vi "interface_configure.vi"(8 "error in (no error)":errorcluster, 11 "config in":T1) -> (0 "error out":errorcluster, 3 "config out":T1)   [LabVIEW 2015, in "lv-builder-l3.lvlib"]
uses:
  lv-builder-l3.lvlib
  _controls/configuration.ctl
  <vilib>/Utility/error.llb/Error Cluster From Error Code.vi
  <vilib>/ErrorRing/Error Ring.xnode
panel:
  in  "cancel":bool
  in  "save":bool
  in  "l3_zip_file_path":path
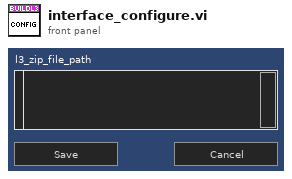
[diagram p1: front panel]
types:
  T1 = typedef "lv-builder-l3.lvlib/configuration.ctl" = cluster{"l3_archive_file_path":string}
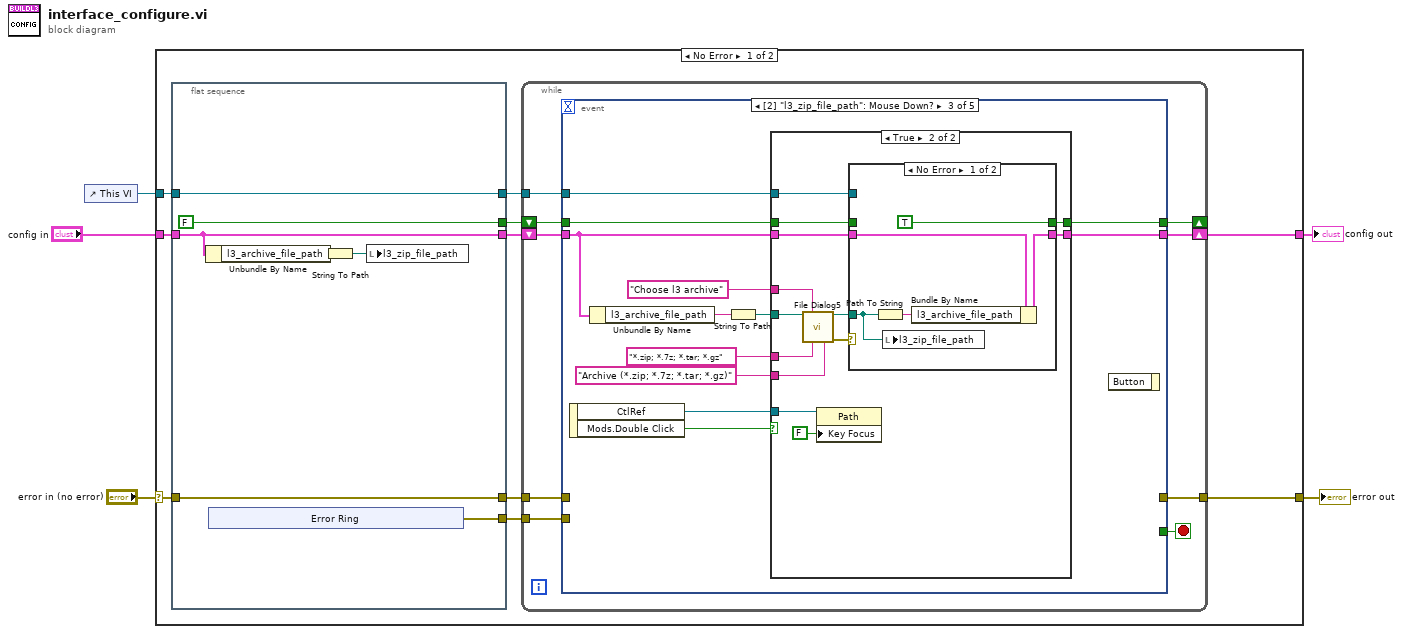
[diagram p0: block diagram]
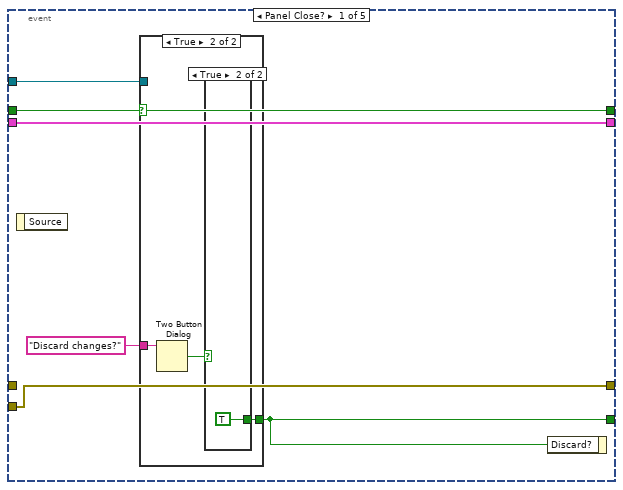
[diagram p2: hidden frame]
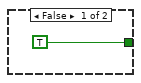
[diagram p3: hidden frame]
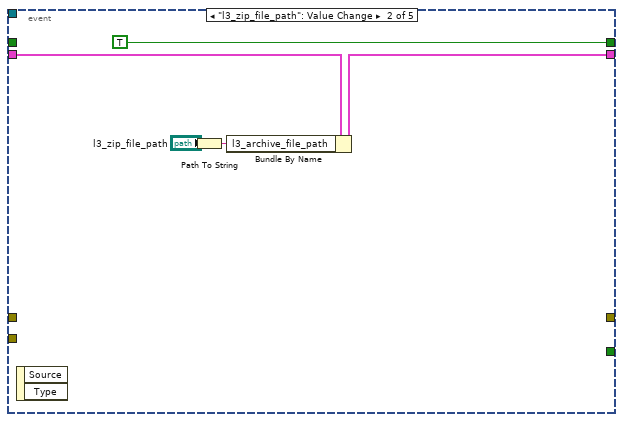
[diagram p5: hidden frame]
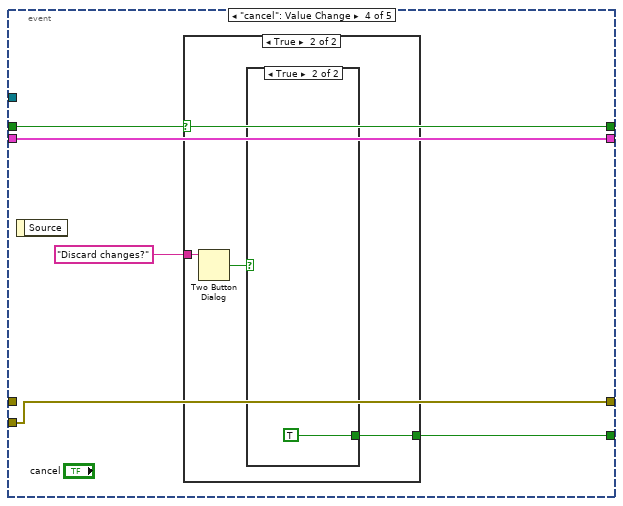
[diagram p8: hidden frame]
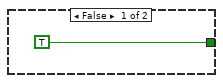
[diagram p9: hidden frame]
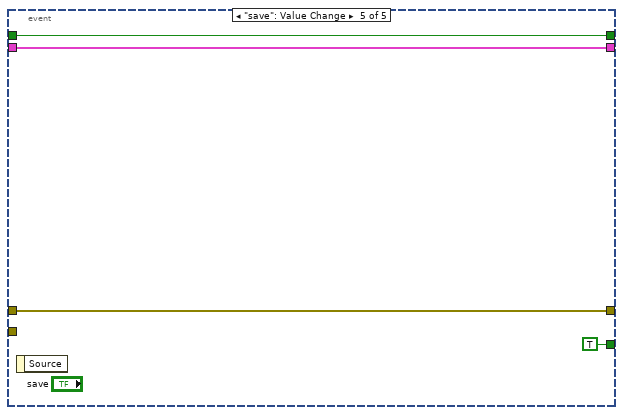
[diagram p11: hidden frame]
diagram:
  n1 = control-ref of="This VI"() -> (w3:refnum<vi>)
  n2 = case shown="No Error" "error in (no error)" {
    selector: "error in (no error)" -> [w15 w100]
    tunnel: [w9 w100] -> w4
    tunnel: w3 -> [w11 _]
    tunnel: [w8 _] -> w2
    tunnel: "config in" -> [w7 _]
    frame No Error {
      n3 = flat-sequence {
        tunnel: w15 -> [w17]
        tunnel: [w17] -> w14
        tunnel: [w18] -> w13
        tunnel: [w20] -> w12
        tunnel: w11 -> [w20]
        tunnel: [FALSE] -> w10
        tunnel: w7 -> [w18]
        tunnel: [w16] -> w6
        frame #0 {
          n4 = Unbundle By Name(w18) -> ("l3_archive_file_path"=w21:string)
          n5 = xnode "Error Ring"() -> ("error out"=w16:errorcluster)
          n6 = String To Path(string=w21) -> (path=w19:path)
          n7 = local write "l3_zip_file_path"(w19) -> ()
        }
      }
      n8 = while {
        tunnel: w14 -> [w28]
        shift-right: [w33] -> w8
        shift-left: w13 -> [w34]
        tunnel: w12 -> [w30]
        shift-right: [w31] -> _
        shift-left: w10 -> [w32]
        tunnel: [w29] -> w9
        tunnel: w6 -> [w27]
        stop <- w35 stop-if-true
        n9 = event shown="[2] \"l3_zip_file_path\": Mouse Down?" {
          selector: _ -> [_ _ _ _ _]
          dyn-events: _ -> [_ _ _ _ _]
          timeout: _ -> [_ _ _ _ _]
          tunnel: [w39 _ _ w90 TRUE ("Discard?")] -> w35
          tunnel: w30 -> [w38 _ w59 _ _]
          tunnel: w34 -> [w41 w51 w58 w89 w98]
          tunnel: [w41 w49 w61 w89 w98] -> w33
          tunnel: w32 -> [w37 _ w63 w87 w99]
          tunnel: [w37 TRUE w62 w87 w99] -> w31
          tunnel: [w36 _ _ w86 w97] -> w29
          tunnel: w28 -> [_ _ _ _ w97]
          tunnel: w27 -> [w36 _ _ w86 _]
          event Panel Close? {
            n10 = event-data() -> ()  [unwired: 1 in, 1 out]
            n11 = case shown="True" w37 {
              tunnel: [TRUE ("Discard?") w45] -> w39
              tunnel: w38 -> [_ _]
              tunnel: "Discard changes?" ("dialog_text") -> [_ w44]
              frame False {
              }
              frame True {
                n12 = Two Button Dialog(message=w44) -> (T button?=w43:bool)  [unwired: 2 in]
                n13 = case shown="True" w43 {
                  tunnel: [_ TRUE ("Discard?")] -> w45
                  frame False {
                  }
                  frame True {
                  }
                }
              }
            }
            n14 = event-data("Discard?"=w39) -> ()  [unwired: 1 in, 1 out]
          }
          event "l3_zip_file_path": Value Change {
            n15 = event-data() -> ()  [unwired: 1 in, 2 out]
            n16 = Path To String(path="l3_zip_file_path") -> (string=w47:string)
            n17 = Bundle By Name(cluster=w51, "l3_archive_file_path"=w47) -> (w49:T1)
          }
          event "l3_zip_file_path": Mouse Down? {
            n18 = event-data() -> ("CtlRef"=w54:refnum<vi>, "Mods.Double Click"=w60:bool)  [unwired: 1 in]
            n19 = Unbundle By Name(w58) -> ("l3_archive_file_path"=w57:string)
            n20 = String To Path(string=w57) -> (path=w55:path)
            n21 = case shown="True" w60 {
              tunnel: w63 -> [w65 w78]
              tunnel: w58 -> [w64 w77]
              tunnel: [w65 w76] -> w62
              tunnel: [w64 w75] -> w61
              tunnel: w59 -> [_ w74]
              tunnel: w55 -> [_ w71]
              tunnel: "Choose l3 archive" ("description") -> [_ w70]
              tunnel: w54 -> [_ w68]
              tunnel: "*.zip; *.7z; *.tar; *.gz" ("pattern (all files)") -> [_ w67]
              tunnel: "Archive (*.zip; *.7z; *.tar; *.gz)" ("pattern label") -> [_ w66]
              frame False {
              }
              frame True {
                n22 = call "File Dialog5"("start path"=w71, "prompt"=w70, "pattern (all files)"=w67, "pattern label"=w66) -> ("selected path"=w72:path, "error out"=w73:errorcluster)  [unwired: 8 in, 2 out]
                n23 = property class="Path"(reference=w68, "Key Focus"=FALSE) -> ()  [unwired: 1 in, 2 out]
                n24 = case shown="No Error" w73 {
                  tunnel: w78 -> [_ w85]
                  tunnel: w77 -> [w82 w84]
                  tunnel: [TRUE w85] -> w76
                  tunnel: [w81 w84] -> w75
                  tunnel: w72 -> [w80 _]
                  tunnel: w74 -> [_ _]
                  frame No Error {
                    n25 = Path To String(path=w80) -> (string=w79:string)
                    n26 = local write "l3_zip_file_path"(w80) -> ()
                    n27 = Bundle By Name(cluster=w82, "l3_archive_file_path"=w79) -> (w81:T1)
                  }
                  frame Error {
                  }
                }
              }
            }
            n28 = event-data() -> ()  [unwired: 2 in, 1 out]
          }
          event "cancel": Value Change {
            n29 = event-data() -> ()  [unwired: 1 in, 1 out]
            n30 = case shown="True" w87 {
              tunnel: [TRUE ("Discard?") w94] -> w90
              tunnel: "Discard changes?" ("dialog_text") -> [_ w92]
              frame False {
              }
              frame True {
                n31 = Two Button Dialog(message=w92) -> (T button?=w93:bool)  [unwired: 2 in]
                n32 = case shown="True" w93 {
                  tunnel: [_ TRUE ("Discard?")] -> w94
                  frame False {
                  }
                  frame True {
                  }
                }
              }
            }
          }
          event "save": Value Change {
            n33 = event-data() -> ()  [unwired: 1 in, 1 out]
          }
        }
      }
    }
    frame Error {
    }
  }
  "error out" <- w4
  "config out" <- w2
